vi "io finder.vi"() -> ()   [LabVIEW 2024]
panel:
  out "return count":u32
  out "find list":string[](array[string])
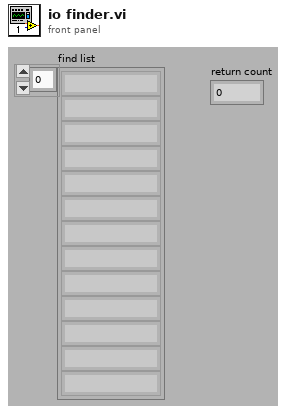
[diagram p1: front panel]
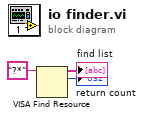
[diagram p0: block diagram]
diagram:
  n1 = VISA Find Resource(11:"?*" ("expression (\"\")")) -> (2:→"return count":u32, 3:→"find list":string[])  [unwired: 2 in, 1 out]
